vi "Reader.vi"(8 "error in (no error)":errorcluster, 10 "Readable":refnum<class "Readable.lvclass">, 11 "Reader in":refnum<class "Reader.lvclass">) -> (0 "error out":errorcluster, 3 "Reader out":refnum<class "Reader.lvclass">)   [LabVIEW 2017, in "Reader.lvclass"]
doc: "Construct a new Reader instance."
uses:
  Reader.lvclass
  Instruments/Utility Classes/Readable/Readable.lvclass
  Reader.lvclass/Reader.ctl
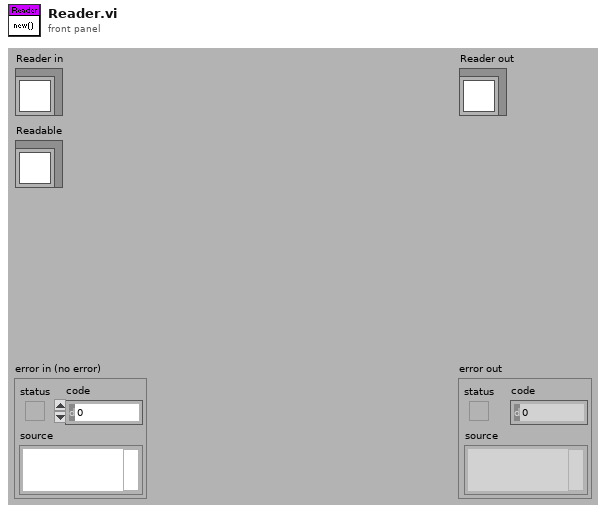
[diagram p1: front panel]
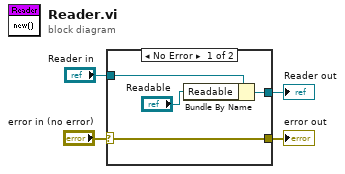
[diagram p0: block diagram]
diagram:
  n1 = case shown="No Error" "error in (no error)" {
    selector: "error in (no error)" -> [w7 w10]
    tunnel: [w7 w10] -> w3
    tunnel: [w6 w9] -> w1
    tunnel: "Reader in" -> [w8 w9]
    frame No Error {
      n2 = Bundle By Name(cluster=w8, "Readable"="Readable") -> (w6:refnum<class "Reader.lvclass">)
    }
    frame Error {
    }
  }
  "error out" <- w3
  "Reader out" <- w1
